vi "Move Timed.vi"(1 "Break on Stop":bool, 2 "Move Speed":dbl=-1.0, 3 "Move Duration (ms)":u32=750) -> ()   [LabVIEW 2013]
panel:
  in  "Move Speed 8":dbl=1.0
  in  "Move Speed 7":dbl=1.0
  in  "Move Speed 6":dbl=1.0
  in  "Move Speed 5":dbl=1.0
  in  "Move Speed 4":dbl=1.0
  in  "Move Speed 3":dbl=1.0
  in  "Move Speed 2":dbl=1.0
  in  "Move Speed":dbl=1.0
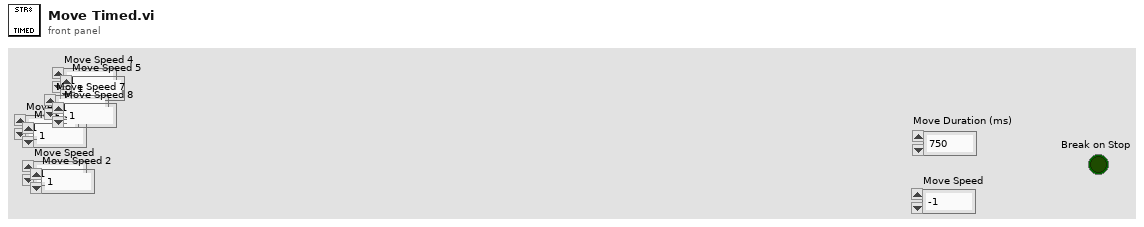
[diagram p1: front panel]
types:
  T1 = typedef "WPI_CounterDevRef.ctl" = cluster{"DevStatus":errorcluster, "CntIndex":T2}
  T2 = typedef "FPGA_CounterCtrSystemIndex.ctl" = enum8{"Ctr 0", "Ctr 1", "Ctr 2", "Ctr 3", "Ctr 4", "Ctr 5", "Ctr 6", "Ctr 7", "Invalid"}
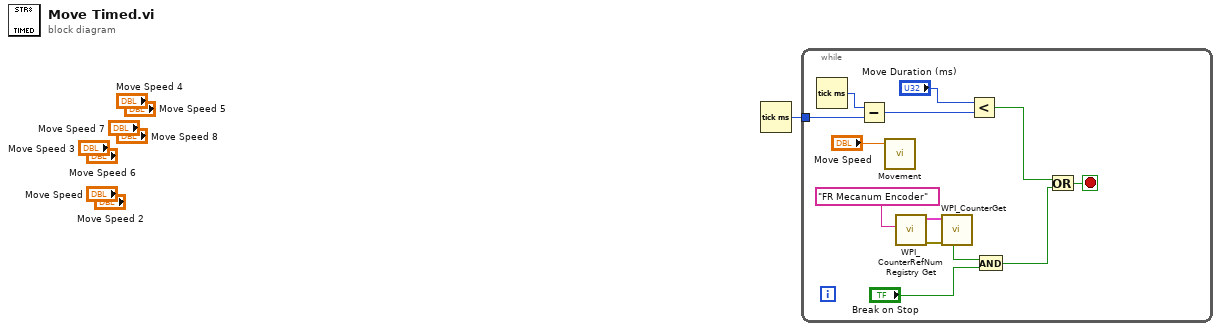
[diagram p0: block diagram]
diagram:
  n1 = Tick Count (ms)() -> (millisecond timer value=w1:u32)
  n2 = while {
    tunnel: w1 -> [w13]
    stop <- w10 stop-if-true
    n3 = Tick Count (ms)() -> (millisecond timer value=w14:u32)
    n4 = Subtract(x=w14, y=w13) -> (x-y=w6:u32)
    n5 = call "Movement.vi"("Forward Speed"="Move Speed") -> ()  [unwired: 2 in]
    n6 = call <vilib>:"WPI_CounterRefNum Registry Get.vi"("refnum name"="FR Mecanum Encoder") -> ("error out"=w9:errorcluster, "CounterDevRef"=w8:T1)  [unwired: 9 in]
    n7 = call <vilib>:"WPI_CounterGet.vi"("error in (no error)"=w9, "CounterDevRef in"=w8) -> ("Stopped"=w2:bool)  [unwired: 4 in, 5 out]
    n8 = Less?(x="Move Duration (ms)", y=w6) -> (x < y?=w5:bool)
    n9 = And(x=w2, y="Break on Stop") -> (x .and. y?=w4:bool)
    n10 = Or(x=w5, y=w4) -> (x .or. y?=w10:bool)
  }
